vi "Read latest Position.vi"(8 "error in (no error)":errorcluster, 11 "Course SIM Motion Axis":refnum<class "Course SIM Motion Axis.lvclass">) -> (0 "error out":errorcluster, 2 "Current Position":dbl, 3 "Course SIM Motion Axis":refnum<class "Course SIM Motion Axis.lvclass">)   [LabVIEW 2022 SP3, in "Course SIM Motion Axis.lvclass"]
uses:
  Course SIM Motion Axis.lvclass
  C:/Stage-Work/XY Stage/Axis Objects/Motion Controller/FINE SIM Motion Axis.lvclass
  Motion Controller/FINE SIM Motion Axis.lvclass/FINE SIM Motion Axis.ctl
  Motion Controller/Accessors/Read Sim Axis Data.vi
  Motion Controller/Accessors/Write Sim Axis Data.vi
  Course SIM Motion Axis.lvclass/Course SIM Motion Axis.ctl
  Motion Controller/FINE SIM Motion Axis.lvclass
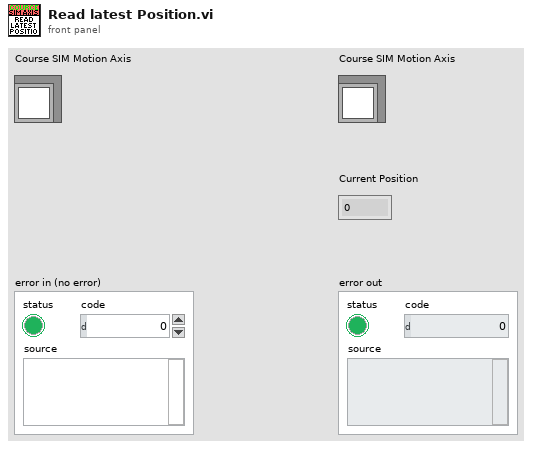
[diagram p1: front panel]
types:
  T1 = typedef "FINE SIM Motion Axis.lvclass/Axis Data.ctl" = cluster{"Axis Parameters":T2, "Time Stamp":timestamp, "Settings":T4}
  T2 = typedef "FINE SIM Motion Axis.lvclass/Axis Parameters.ctl" = cluster{"Moving":bool, "Homed":bool, "Desired Position":dbl, "Current Positon":dbl, "Current Speed":dbl, "Home Status":T3}
  T3 = typedef "FINE SIM Motion Axis.lvclass/Homing Status.ctl" = enum16{"Idle", "Inital Home Motion", "Final Home Motion", "Done Homing"}
  T4 = typedef "FINE SIM Motion Axis.lvclass/Settings.ctl" = cluster{"Axis Name":string, "Axis Settings":T5}
  T5 = typedef "FINE SIM Motion Axis.lvclass/Axis Settings.ctl" = cluster{"Speed":dbl, "Acceleration":dbl}
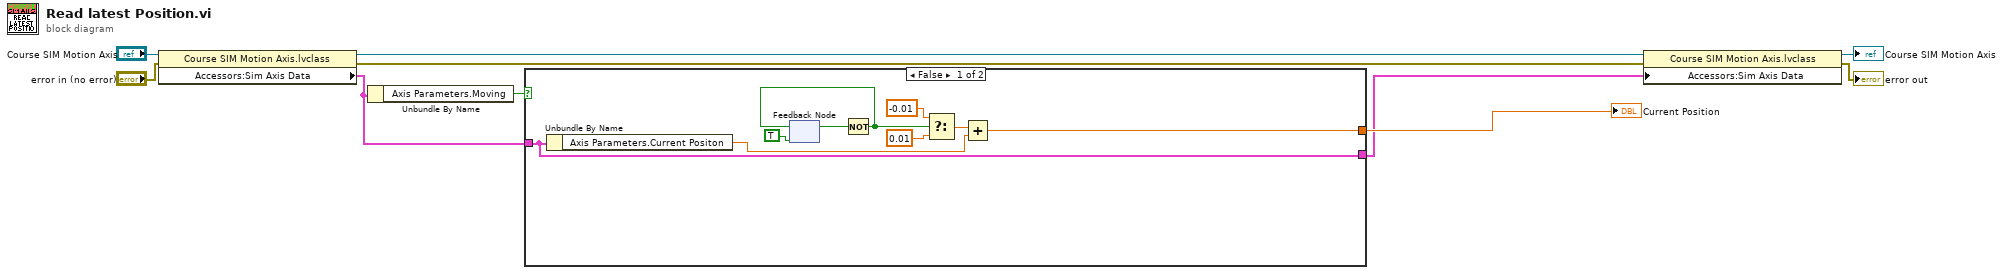
[diagram p0: block diagram]
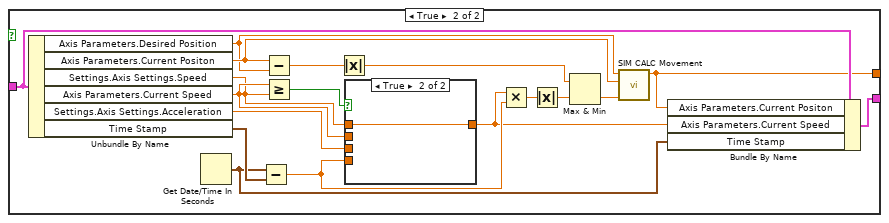
[diagram p2: hidden frame]
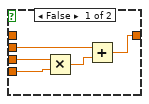
[diagram p3: hidden frame]
diagram:
  n1 = property class="Course SIM Motion Axis.lvclass"(reference="Course SIM Motion Axis", error in="error in (no error)") -> (reference out=w4:refnum<class "Course SIM Motion Axis.lvclass">, error out=w3:errorcluster, "Accessors:Sim Axis Data"=w1:T1)
  n2 = Unbundle By Name(w1) -> ("Axis Parameters.Moving"=w2:bool)
  n3 = case shown="False" w2 {
    tunnel: w1 -> [w19 w37]
    tunnel: [w19 w35] -> w5
    tunnel: [w12 w36] -> w9
    frame False {
      n4 = Unbundle By Name(w19) -> ("Axis Parameters.Current Positon"=w11:dbl)
      n5 = feedback #1(TRUE) -> (w17:bool)
      n6 = Not(x=w17) -> (.not. x?=w16:bool)
      n7 = feedback-in #1(w16) -> ()
      n8 = Select(t=-0.01 ("f"), s=w16, f=0.01) -> (s? t:f=w13:dbl)
      n9 = Add(x=w13, y=w11) -> (x+y=w12:dbl)
    }
    frame True {
      n10 = Unbundle By Name(w37) -> ("Axis Parameters.Desired Position"=w26:dbl, "Axis Parameters.Current Positon"=w27:dbl, "Settings.Axis Settings.Speed"=w20:dbl, "Axis Parameters.Current Speed"=w32:dbl, "Settings.Axis Settings.Acceleration"=w31:dbl, "Time Stamp"=w29:timestamp)
      n11 = Get Date/Time In Seconds() -> (seconds since 1Jan1904=w28:timestamp)
      n12 = Subtract(x=w28, y=w29) -> (x-y=w34:dbl)
      n13 = Subtract(x=w27, y=w26) -> (x-y=w25:dbl)
      n14 = Greater Or Equal?(x=w32, y=w20) -> (x >= y?=w33:bool)
      n15 = Absolute Value(x=w25) -> (abs(x)=w23:dbl)
      n16 = case shown="True" w33 {
        tunnel: [w38 w43] -> w30
        tunnel: w32 -> [w39 _]
        tunnel: w34 -> [w42 _]
        tunnel: w31 -> [w41 _]
        tunnel: w20 -> [_ w43]
        frame False {
          n17 = Multiply(x=w41, y=w42) -> (x*y=w40:dbl)
          n18 = Add(x=w39, y=w40) -> (x+y=w38:dbl)
        }
        frame True {
        }
      }
      n19 = Multiply(x=w30, y=w34) -> (x*y=w24:dbl)
      n20 = Absolute Value(x=w24) -> (abs(x)=w22:dbl)
      n21 = Max & Min(x=w23, y=w22) -> (min(x,y)=w21:dbl)  [unwired: 1 out]
      n22 = call "SIM CALC Movement.vi"("New Distance"=w21, "Current"=w27, "Desired"=w26) -> ("New Current"=w36:dbl)  [unwired: 8 in]
      n23 = Bundle By Name(cluster=w37, "Axis Parameters.Current Positon"=w36, "Axis Parameters.Current Speed"=w30, "Time Stamp"=w28) -> (w35:T1)
    }
  }
  "Current Position" <- w9
  n24 = property class="Course SIM Motion Axis.lvclass"(reference=w4, error in=w3, "Accessors:Sim Axis Data"=w5) -> (reference out=→"Course SIM Motion Axis":refnum<class "Course SIM Motion Axis.lvclass">, error out=→"error out":errorcluster)
